vi "RT Finialize.vi"(8 "error in (no error)":errorcluster, 11 "RT Data Cluster in":T1={"Timekeeper hdl"="", "clkDisc session"=variant, "Compiled Data"={"SyncMod?"=FALSE, "SyncMod"="", "ConnectionSettings"={"Mode"=enum."Generate sample clock", "pxitrig"=FALSE, "pfi0"=FALSE, "pfi1"=FALSE, "pfi2"=FALSE, "External Pin"=enum."PFI0", "Routes"=[]}, "TimeKeeper"="", "ScanOffset(%)"=0.0, "StartDelay(s)"=0, "Time Ref Settings"={"Time Reference"=enum."GPS", "Priority 1"=0, "Priority 2"=0, "IRIG type"=enum."IRIGB AM", "Terminal"="", "PPSSetTime"=FALSE, "Start Time"=timestamp(0 s since 1904-01-01)}, "FIFO Locations"={"BoardTime"=[], "Status"=[]}}, "OutputsData"=[], "OutputsFIFO"=refnum, "Scan Period"=0, "Timekeeper type"=enum."6683", "SyncMod type"=enum."6683", "SyncMod hdl"=""} {"Compiled Data"."Time Ref Settings"."Priority 2" min=0 max=255; "Compiled Data"."Time Ref Settings"."Priority 1" min=0 max=255}) -> (0 "error out":errorcluster)   [LabVIEW 2015, in "Chassis TimeSync Engine.lvlib"]
uses:
  Chassis TimeSync Engine.lvlib
  RT Data Cluster.ctl
  mdevClkDisc.llb/_clkDisc_session.ctl
  Shared/Compiled Data.ctl
  Shared/Connection Settings.ctl
  Shared/Mode.ctl
  Shared/External Pin.ctl
  Shared/Routes.ctl
  Shared/Route.ctl
  Shared/Time Ref Settings.ctl
  Shared/Time Reference.ctl
  Shared/IRIG Type.ctl
  timekeeper type.ctl
  Shared/Chassis TimeSync Shared.lvlib
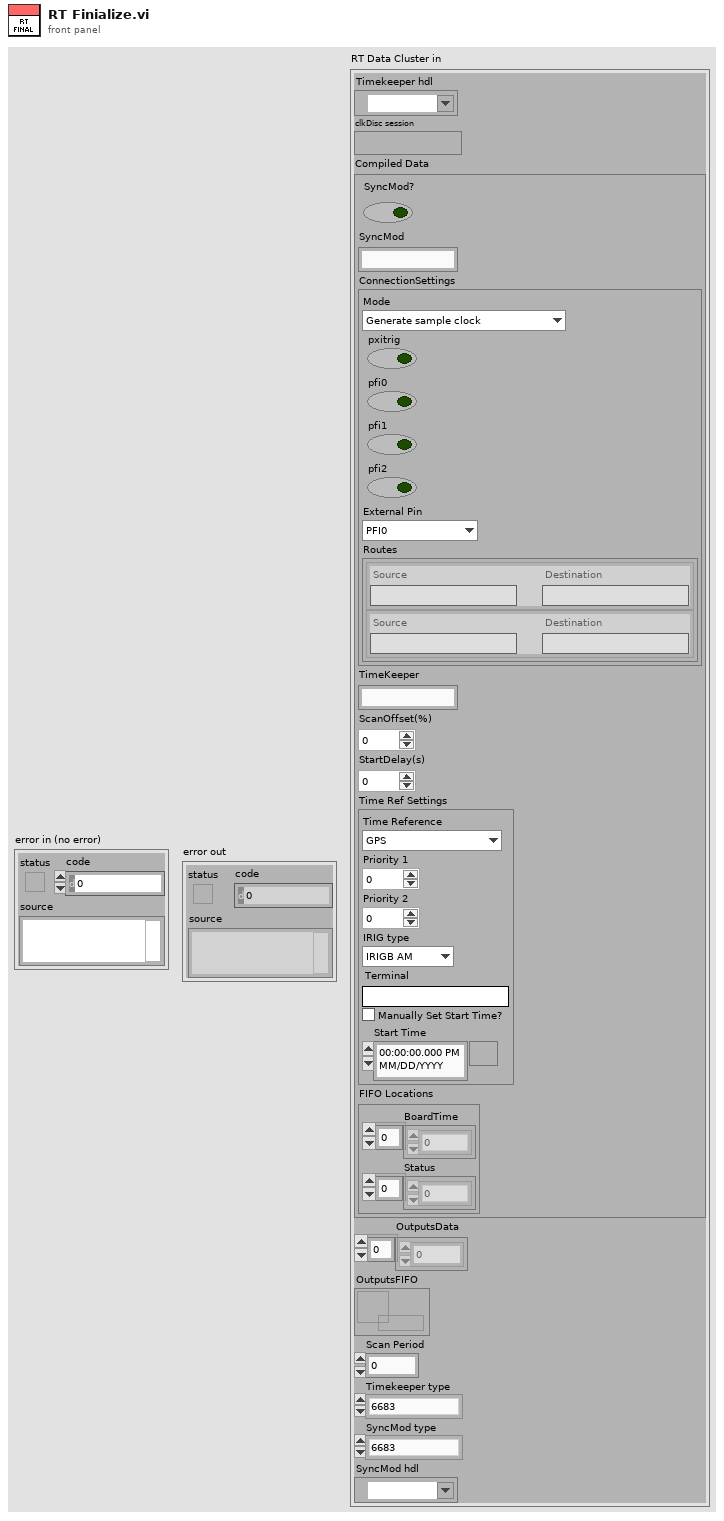
[diagram p1: front panel]
types:
  T1 = typedef "Chassis TimeSync Engine.lvlib/RT Data Cluster.ctl" = cluster{"Timekeeper hdl":refnum<k15>, "clkDisc session":T2, "Compiled Data":T3, "OutputsData":dbl[], "OutputsFIFO":refnum<k33>, "Scan Period":u32, "Timekeeper type":T12, "SyncMod type":T12, "SyncMod hdl":refnum<k15>}
  T2 = typedef "_clkDisc_session.ctl" = variant
  T3 = typedef "Chassis TimeSync Shared.lvlib/Compiled Data.ctl" = cluster{"SyncMod?":bool, "SyncMod":string, "ConnectionSettings":T4, "TimeKeeper":string, "ScanOffset(%)":dbl, "StartDelay(s)":u16, "Time Ref Settings":T9, "FIFO Locations":cluster{"BoardTime":i32[], "Status":i32[]}}
  T4 = typedef "Chassis TimeSync Shared.lvlib/Connection Settings.ctl" = cluster{"Mode":T5, "pxitrig":bool, "pfi0":bool, "pfi1":bool, "pfi2":bool, "External Pin":T6, "Routes":T7}
  T5 = typedef "Chassis TimeSync Shared.lvlib/Mode.ctl" = enum16{"Generate sample clock", "Route sample clock out of chassis", "Route sample clock into chassis", "Custom routes"}
  T6 = typedef "Chassis TimeSync Shared.lvlib/External Pin.ctl" = enum16{"PFI0", "PFI1", "PFI2"}
  T7 = typedef "Chassis TimeSync Shared.lvlib/Routes.ctl" = T8[]
  T8 = typedef "Chassis TimeSync Shared.lvlib/Route.ctl" = cluster{"Source":string, "Destination":string}
  T9 = typedef "Chassis TimeSync Shared.lvlib/Time Ref Settings.ctl" = cluster{"Time Reference":T10, "Priority 1":i32, "Priority 2":i32, "IRIG type":T11, "Terminal":string, "PPSSetTime":bool, "Start Time":timestamp}
  T10 = typedef "Chassis TimeSync Shared.lvlib/Time Reference.ctl" = enum16{"GPS", "IRIG", "PPS", "1588 Ordinary Clock", "PXI Chassis Clock", "Free Running (Internal)"}
  T11 = typedef "Chassis TimeSync Shared.lvlib/IRIG Type.ctl" = enum16{"IRIGB DC", "IRIGB AM"}
  T12 = typedef "Chassis TimeSync Engine.lvlib/timekeeper type.ctl" = enum16{"6683", "6683H", "6682", "6682H", "non-timekeeper", "timekeeper"}
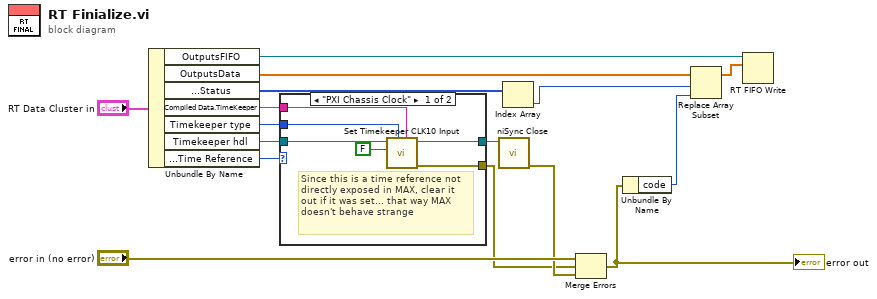
[diagram p0: block diagram]
diagram:
  n1 = Unbundle By Name("RT Data Cluster in") -> ("OutputsFIFO"=w10:refnum<k33>, "OutputsData"=w12:dbl[], "Compiled Data.FIFO Locations.Status"=w13:i32[], "Compiled Data.TimeKeeper"=w1:string, "Timekeeper type"=w2:T12, "Timekeeper hdl"=w5:refnum<k15>, "Compiled Data.Time Ref Settings.Time Reference"=w6:T10)
  n2 = case shown="\"PXI Chassis Clock\"" w6 {
    tunnel: w5 -> [w21 w23]
    tunnel: [w20 w23] -> w4
    tunnel: [w22 _] -> w3
    tunnel: w2 -> [w18 _]
    tunnel: w1 -> [w17 _]
    frame "PXI Chassis Clock" {
      # "Since this is a time reference not directly exposed in MAX, clear it out if it was set... that way MAX doesn't behave strange"
      n3 = call "Set Timekeeper CLK10 Input.vi"("Timekeeper"=w17, "Timekeeper type"=w18, "Enabled?"=FALSE ("Advanced:Time Reference:Clk10 Disciplining Enabled"), "timekeeper in"=w21) -> ("error out"=w22:errorcluster, "timekeeper out"=w20:refnum<k15>)  [unwired: 6 in]
    }
    frame Default {
    }
  }
  n4 = call <instrlib>:"niSync Close.vi"("instrument handle"=w4) -> ("error out"=w14:errorcluster)  [unwired: 10 in]
  n5 = Index Array(array=w13) -> (element=w11:i32)  [unwired: 1 in]
  n6 = Merge Errors("error in (no error)", w3, w14) -> (w7:errorcluster)
  "error out" <- w7
  n7 = Unbundle By Name(w7) -> ("code"=w8:i32)
  n8 = Replace Array Subset(array=w12, new element=w8, index=w11) -> (w9:dbl[])
  n9 = RT FIFO Write(0:w10, 1:w9) -> ()  [unwired: 3 in, 4 out]
